vi "CRYCalc Result item.vi"(5 "Statistic Run Number":i32, 6 "Step Setup VI No":i32, 7 "Statistic Item":T4(ring), 8 "+/-Adjust(Deviation)":i32, 9 "Work in":u16, 10 "Results in":T2 {"Margin" format="%.2f"}) -> (3 "Result  run Out":T1[](array[typedef]) {"Z data" items=["dB", "Lin"]; "X data" items=["dB", "Lin"]; "Y data" items=["dB", "Lin"]; "Z dB ref" format="%.1f"; "Z axis" items=["Log", "Lin"]; "X dB ref" format="%.1f"; "X axis" items=["Log", "Lin"]; "Y axis" items=["Log", "Lin"]; "Y dB ref" format="%.1f"; "Curve"."z" format="%.2f"; "Curve"."y" format="%.2f"; "Curve"."x" format="%.2f"})   [LabVIEW 2013]
uses:
  Typedef Control/CRYResult Cluster Array.ctl
  Typedef Control/CRYResult Cluster.ctl
  Typedef Control/CRYData Cluster.ctl
  CRYStatistics Global.vi
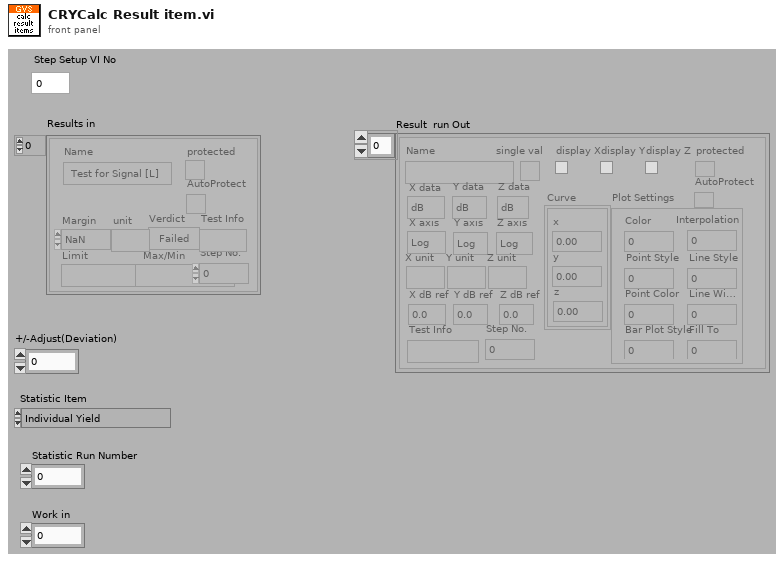
[diagram p1: front panel]
types:
  T1 = typedef "CRYData Cluster.ctl" = cluster{"Name":string, "Curve":cluster{"x":dbl, "y":dbl, "z":dbl}[], "X data":u16, "Y data":u16, "Z data":u16, "X axis":u16, "Y axis":u16, "Z axis":u16, "X unit":string, "Y unit":string, "Z unit":string, "X dB ref":dbl, "Y dB ref":dbl, "Z dB ref":dbl, "single val":bool, "protected":bool, "display X":bool, "display Y":bool, "display Z":bool, "Test Info":string, "Step No.":i32, "Plot Settings":cluster{"Color":u32, "Interpolation":u8, "Point Style":u8, "Line Style":u8, "Point Color":u32, "Line Width":u8, "Bar Plot Style":u8, "Fill To":i16}, "AutoProtect":bool}
  T2 = typedef "CRYResult Cluster Array.ctl" = T3[]
  T3 = typedef "CRYResult Cluster.ctl" = cluster{"Name":string, "Margin":dbl, "unit":string, "Verdict":bool, "Limit":string, "Max/Min":string, "protected":bool, "Step No.":i32, "Test Info":string, "AutoProtect":bool}
  T4 = enum32{"Individual Yield", "Overall Yield", "Mean", "Absolute Standard Deviation", "Standard Deviation"}
  T5 = typedef "CRYData Cluster Array.ctl" = T1[]
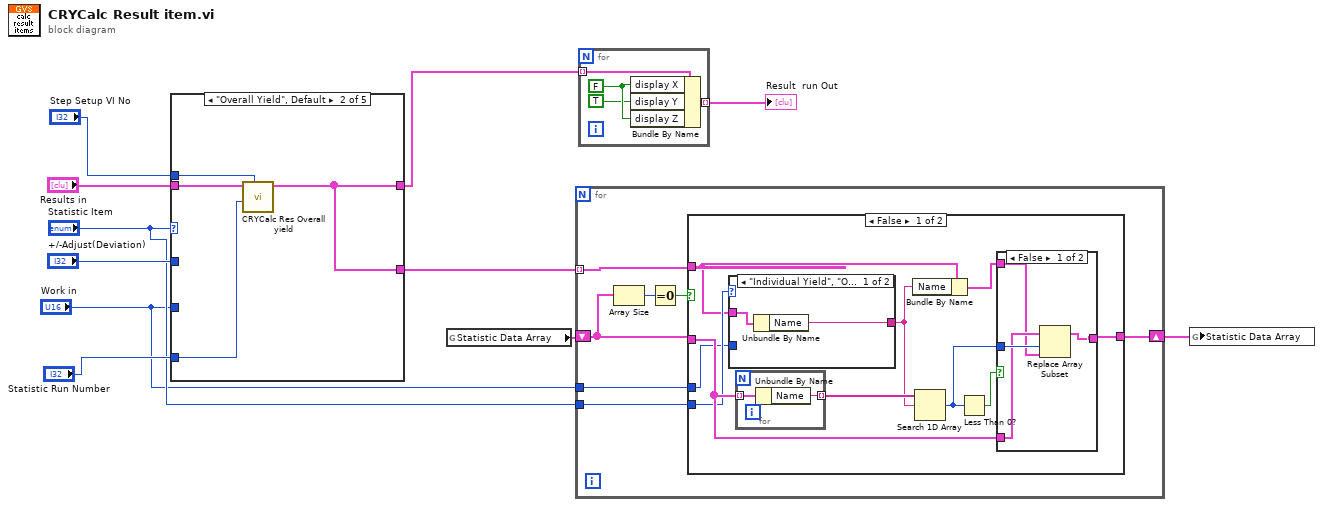
[diagram p0: block diagram]
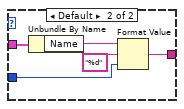
[diagram p2: hidden frame]
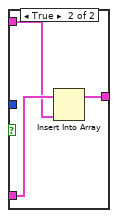
[diagram p3: hidden frame]
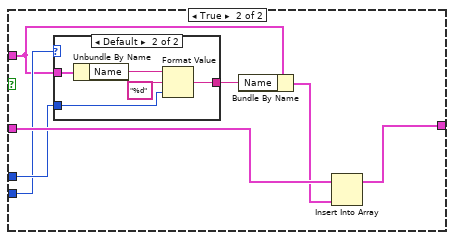
[diagram p4: hidden frame]
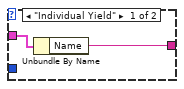
[diagram p5: hidden frame]
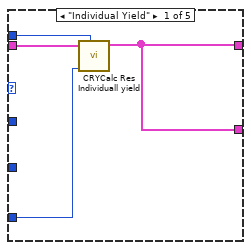
[diagram p6: hidden frame]
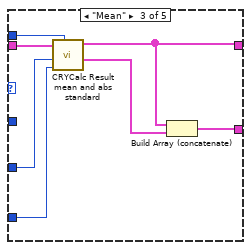
[diagram p7: hidden frame]
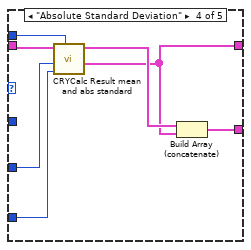
[diagram p8: hidden frame]
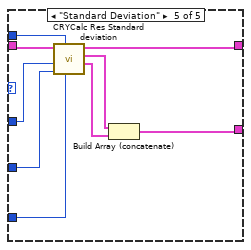
[diagram p9: hidden frame]
diagram:
  n1 = case shown="\"Overall Yield\", Default" "Statistic Item" {
    tunnel: "Results in" -> [w15 w19 w26 w30 w37]
    tunnel: [w14 w17 w25 w32 w39] -> w9
    tunnel: "+/-Adjust(Deviation)" -> [_ _ _ _ w36]
    tunnel: [w14 w17 w23 w31 w40] -> w5
    tunnel: "Step Setup VI No" -> [w13 w18 w22 w29 w38]
    tunnel: "Statistic Run Number" -> [w12 w16 w21 w28 w35]
    tunnel: "Work in" -> [_ _ w20 w27 w34]
    frame "Individual Yield" {
      n2 = call "CRYCalc Res Individuall yield.vi"("Step Setup VI No"=w13, "Statistic Run Number"=w12, "Results in"=w15) -> ("Individuall Yield Out"=w14:T1[])  [unwired: 8 in]
    }
    frame "Overall Yield", Default {
      n3 = call "CRYCalc Res Overall yield.vi"("Step Setup VI No"=w18, "Statistic Run Number"=w16, "Results in"=w19) -> ("Overall Yield Out"=w17:T1[])  [unwired: 1 in, 7 out]
    }
    frame "Mean" {
      n4 = call "CRYCalc Result mean and abs standard.vi"("Step Setup VI No"=w22, "Statistic Run Number"=w21, "Work in"=w20, "Results in"=w26) -> ("Margin Std Dev Out"=w24:T1[], "Margin mean Out"=w25:T1[])  [unwired: 1 in, 5 out]
      n5 = Build Array (concatenate)(w25, w24) -> (w23:T1[])
    }
    frame "Absolute Standard Deviation" {
      n6 = call "CRYCalc Result mean and abs standard.vi"("Step Setup VI No"=w29, "Statistic Run Number"=w28, "Work in"=w27, "Results in"=w30) -> ("Margin Std Dev Out"=w32:T1[], "Margin mean Out"=w33:T1[])  [unwired: 5 in, 1 out]
      n7 = Build Array (concatenate)(w33, w32) -> (w31:T1[])
    }
    frame "Standard Deviation" {
      n8 = call "CRYCalc Res Standard deviation.vi"("Statistic Run Number"=w35, "Step Setup VI No"=w38, "Work in"=w34, "+/-Adjust(Deviation)"=w36, "Results in"=w37) -> ("Margin Std Dev Out"=w42:T1[], "Margin mean Out"=w41:T1[], "Standard Dev Out"=w39:T1[])  [unwired: 1 in, 3 out]
      n9 = Build Array (concatenate)(w41, w42) -> (w40:T1[])
    }
  }
  n10 = global read "CRYStatistics Global.vi" "Statistic Data Array"() -> (w7:T5)
  n11 = for {
    tunnel: w5 -> [w45] mode=indexing
    shift-right: [w47] -> w6
    shift-left: w7 -> [w46]
    tunnel: "Statistic Item" -> [w44]
    tunnel: "Work in" -> [w43]
    n12 = Array Size(array=w46) -> (size(s)=w49:i32)
    n13 = Equal To 0?(x=w49) -> (x = 0?=w48:bool)
    n14 = case shown="False" w48 {
      tunnel: [w56 w82] -> w47
      tunnel: w46 -> [w57 w81]
      tunnel: w45 -> [w52 w77]
      tunnel: w44 -> [w54 w79]
      tunnel: w43 -> [w53 w80]
      frame False {
        n15 = case shown="\"Individual Yield\", \"Overall Yield\"" w54 {
          tunnel: [w60 w62] -> w51
          tunnel: w52 -> [w61 w66]
          tunnel: w53 -> [_ w63]
          frame "Individual Yield", "Overall Yield" {
            n16 = Unbundle By Name(w61) -> ("Name"=w60:string)
          }
          frame Default {
            n17 = Unbundle By Name(w66) -> ("Name"=w64:string)
            n18 = Format Value(string ("")=w64, format string="%d", value (0)=w63) -> (output string=w62:string)
          }
        }
        n19 = for {
          tunnel: w57 -> [w75] mode=indexing
          tunnel: [w74] -> w59 mode=indexing
          n20 = Unbundle By Name(w75) -> ("Name"=w74:string)
        }
        n21 = Bundle By Name(cluster=w52, "Name"=w51) -> (w50:T1)
        n22 = Search 1D Array(1D array=w59, element=w51) -> (index of element=w55:i32)  [unwired: 1 in]
        n23 = Less Than 0?(x=w55) -> (x < 0?=w58:bool)
        n24 = case shown="False" w58 {
          tunnel: w57 -> [w69 w73]
          tunnel: w50 -> [w68 w72]
          tunnel: [w67 w71] -> w56
          tunnel: w55 -> [w70 _]
          frame False {
            n25 = Replace Array Subset(array=w69, new element=w68, index=w70) -> (w67:T5)
          }
          frame True {
            n26 = Insert Into Array(array=w73, new element=w72) -> (w71:T5)  [unwired: 1 in]
          }
        }
      }
      frame True {
        n27 = case shown="Default" w79 {
          tunnel: [w83 w85] -> w78
          tunnel: w77 -> [w84 w89]
          tunnel: w80 -> [_ w86]
          frame "Individual Yield" {
            n28 = Unbundle By Name(w84) -> ("Name"=w83:string)
          }
          frame Default {
            n29 = Unbundle By Name(w89) -> ("Name"=w87:string)
            n30 = Format Value(string ("")=w87, format string="%d", value (0)=w86) -> (output string=w85:string)
          }
        }
        n31 = Bundle By Name(cluster=w77, "Name"=w78) -> (w76:T1)
        n32 = Insert Into Array(array=w81, new element=w76) -> (w82:T5)  [unwired: 1 in]
      }
    }
  }
  n33 = for {
    tunnel: w9 -> [w93] mode=indexing
    tunnel: [w92] -> w8 mode=indexing
    w91 = FALSE ("display X")
    n34 = Bundle By Name(cluster=w93, "display X"=w91, "display Y"=TRUE, "display Z"=w91) -> (w92:T1)
  }
  "Result  run Out" <- w8
  n35 = global write "CRYStatistics Global.vi" "Statistic Data Array"(w6) -> ()
